vi "Init Item.vi"(5 "Item Update":refnum<user-event>, 7 "Blueprint":refnum<class "Blueprint.lvclass">, 8 "error in (no error)":errorcluster, 9 "Removable? (F)":bool, 10 "Qty":i32, 11 "Item":refnum<class "Item.lvclass">) -> (0 "error out":errorcluster, 3 "BP Item out":refnum<class "BP Item.lvclass">)   [LabVIEW 2020, in "BP Item.lvclass"]
uses:
  BP Item.lvclass
  Item/Item.lvclass
  Blueprint/Blueprint.lvclass
  Item/Ingredient.ctl
  BP Item.lvclass/BP Item.ctl
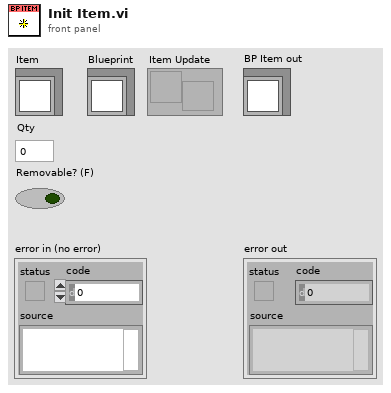
[diagram p1: front panel]
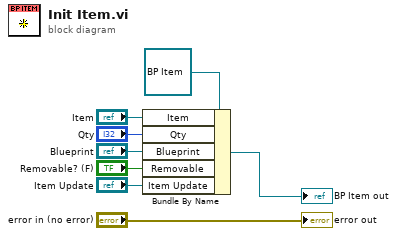
[diagram p0: block diagram]
diagram:
  n1 = Bundle By Name(cluster=refnum<class "BP Item.lvclass"> refnum ("BP Item in"), "Item"="Item", "Qty"="Qty", "Blueprint"="Blueprint", "Removable"="Removable? (F)", "Item Update"="Item Update") -> (→"BP Item out":refnum<class "BP Item.lvclass">)
  "error out" <- "error in (no error)"
